vi "PlotCenterIR.vi"(1 "StepAngle":i32, 2 "IR_D":dbl, 3 "InWorld":i16[][](array[numeric])) -> (0 "OutWorld":i16[][](graph))   [LabVIEW 2014]
panel:
  out "InWorld":i16[][](graph)
  out "OutWorld":i16[][](array[numeric])
  out "Pixel 2":i16
  out "X Pixel":i16
  out "Y Pixel":i16
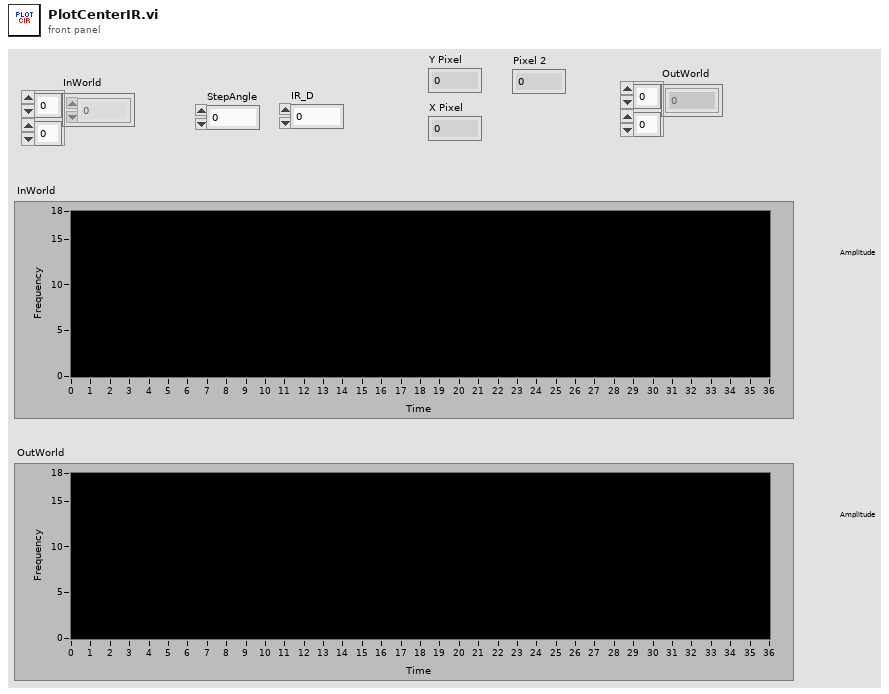
[diagram p1: front panel]
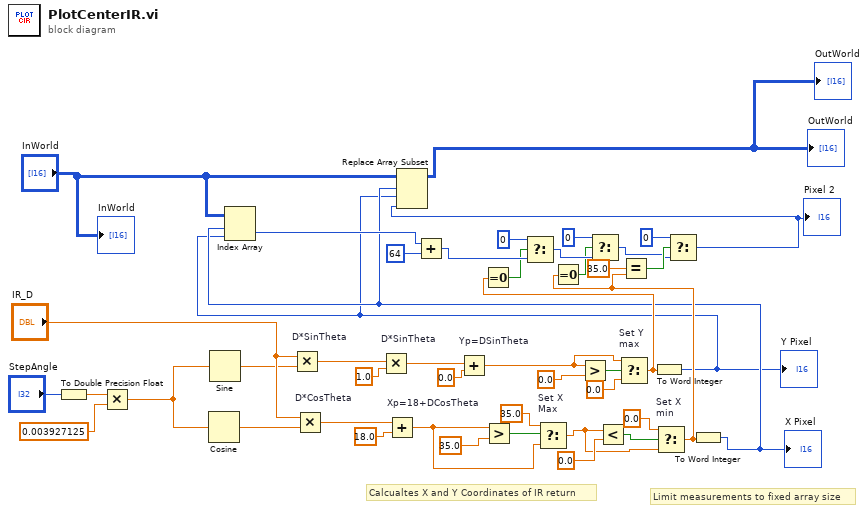
[diagram p0: block diagram]
diagram:
  # "Limit measurements to fixed array size"
  # "Calcualtes X and Y Coordinates of IR return"
  n1 = To Double Precision Float(number="StepAngle") -> (double precision float=w43:dbl)
  n2 = Multiply(x=w43, y=0.003927125) -> (x*y=w41:dbl)
  n3 = Cosine(x=w41) -> (cos(x)=w38:dbl)
  n4 = Sine(x=w41) -> (sin(x)=w39:dbl)
  n5 = Multiply "D*SinTheta"(x="IR_D", y=w39) -> (x*y=w37:dbl)
  n6 = Multiply "D*CosTheta"(x="IR_D", y=w38) -> (x*y=w35:dbl)
  n7 = Multiply "D*SinTheta"(x=w37, y=1.0) -> (x*y=w33:dbl)
  n8 = Add "Xp=18+DCosTheta"(x=w35, y=18.0) -> (x+y=w29:dbl)
  n9 = Add "Yp=DSinTheta"(x=w33, y=0.0) -> (x+y=w20:dbl)
  n10 = Greater?(x=w29, y=35.0) -> (0:w30:bool)
  n11 = Select "Set X \nMax"(t=35.0, s=w30, f=w29) -> (s? t:f=w24:dbl)
  n12 = Greater?(x=w20, y=0.0) -> (0:w22:bool)
  n13 = Less?(x=w24, y=0.0) -> (x < y?=w25:bool)
  n14 = Select "Set Y \nmax"(t=w20, s=w22, f=0.0) -> (s? t:f=w14:dbl)
  n15 = Equal To 0?(x=w14) -> (x = 0?=w15:bool)
  n16 = To Word Integer(number=w14) -> (16bit integer=w1:i16)
  "Y Pixel" <- w1
  n17 = Select "Set X\nmin"(t=0.0, s=w25, f=w24) -> (s? t:f=w8:dbl)
  n18 = Equal To 0?(x=w8) -> (x = 0?=w10:bool)
  n19 = Equal?(x=35.0, y=w8) -> (x = y?=w9:bool)
  n20 = To Word Integer(number=w8) -> (16bit integer=w2:i16)
  "X Pixel" <- w2
  n21 = Index Array "Index Array"(array="InWorld", index (row)=w2, index (col)=w1) -> (element=w17:i16)
  n22 = Add(x=w17, y=i16 64) -> (x+y=w16:i16)
  n23 = Select(t=i16 0, s=w15, f=w16) -> (s? t:f=w13:i16)
  n24 = Select(t=i16 0, s=w10, f=w13) -> (s? t:f=w5:i16)
  n25 = Select(t=i16 0, s=w9, f=w5) -> (s? t:f=w4:i16)
  "Pixel 2" <- w4
  n26 = Replace Array Subset(array="InWorld", new element=w4, index (row)=w2, index (col)=w1) -> (→"OutWorld" →"OutWorld":i16[][])
  "InWorld" <- "InWorld"
